vi "start.vi"(8 "error in (no error)":errorcluster, 11 "DL090202ScanHead in":refnum<class "ScanHeadDL090202.lvclass">) -> (0 "error out":errorcluster, 3 "DL090202ScanHead out":refnum<class "ScanHeadDL090202.lvclass">)   [LabVIEW 2010, in "ScanHeadDL090202.lvclass"]
uses:
  ScanHeadDL090202.lvclass
  SignalWriter/GenericSignalWriter/GenericSignalWriter/GenericSignalWriter.lvclass
  DAQ/GenericDAQ/GenericDAQ/GenericDAQ.lvclass
  Trajectory/GenericTrajectory/GenericTrajectory/GenericTrajectory.lvclass
  Clock/GenericClock/GenericClock/GenericClock.lvclass
  common/classes/ErrorController/ErrorController/ErrorController.lvclass
  DigitalOut/GenericDigitalOut/GenericDigitalOut/GenericDigitalOut.lvclass
  common/classes/GenericComponent/GenericComponent/GenericComponent.lvclass
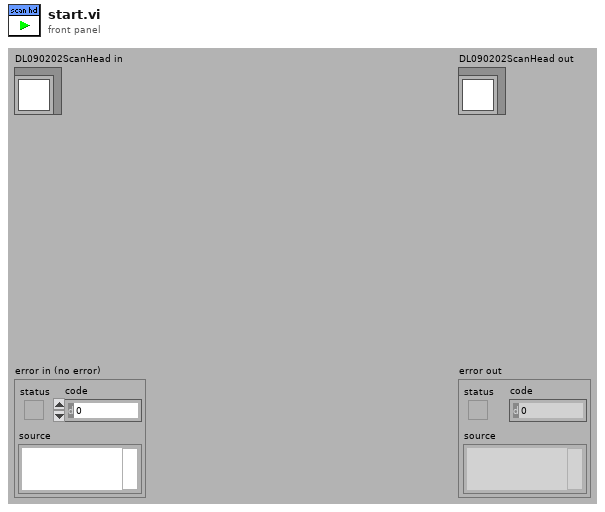
[diagram p1: front panel]
types:
  T1 = typedef "GenericToplevelComponent.lvclass/common_trigger_enum.ctl" = enum16{"NULL", "initialise", "terminate", "fetch command", "fetch data", "attach observer", "register as observer", "detach observer", "acknowledge", "start", "stop", "sweep started", "sweep finished", "experiment started", "experiment stopped"}
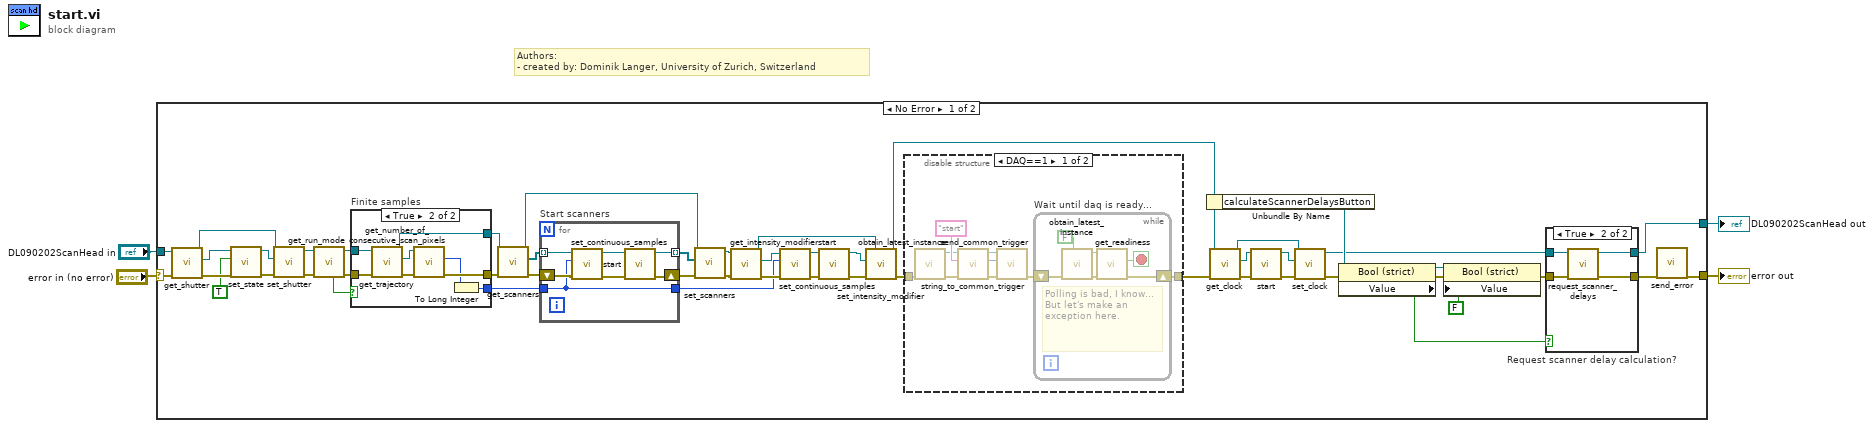
[diagram p0: block diagram]
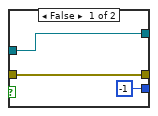
[diagram p4: hidden frame]
diagram:
  # "Authors: \n- created by: Dominik Langer, University of Zurich, Switzerland"
  n1 = case shown="No Error" "error in (no error)" {
    selector: "error in (no error)" -> [w21 w96]
    tunnel: [w10 w96] -> w3
    tunnel: [w5 w95] -> w1
    tunnel: "DL090202ScanHead in" -> [w22 w95]
    frame No Error {
      n2 = call-dynamic "get_shutter.vi"("error in (no error)"=w21, "DL090202ScanHead.lvclass in"=w22) -> ("error out"=w54:errorcluster, "GenericDigitalOut.lvclass"=w52:refnum<class "GenericDigitalOut.lvclass">, "DL090202ScanHead.lvclass out"=w51:refnum<class "ScanHeadDL090202.lvclass">)  [unwired: 7 out]
      n3 = call-dynamic "set_state.vi"("error in (no error)"=w54, "state"=TRUE, "GenericDigitalOut in"=w52) -> ("error out"=w53:errorcluster, "GenericDigitalOut out"=w50:refnum<class "GenericDigitalOut.lvclass">)  [unwired: 7 in]
      n4 = call-dynamic "set_shutter.vi"("error in (no error)"=w53, "GenericDigitalOut.lvclass"=w50, "DL090202ScanHead.lvclass in"=w51) -> ("error out"=w28:errorcluster, "DL090202ScanHead.lvclass out"=w29:refnum<class "ScanHeadDL090202.lvclass">)  [unwired: 7 out]
      n5 = call "get_run_mode.vi"("error in (no error)"=w28, "GenericPlugin in"=w29) -> ("error out"=w27:errorcluster, "GenericPlugin out"=w26:refnum<class "ScanHeadDL090202.lvclass">, "is NOT free run?"=w25:bool)  [unwired: 5 in, 2 out]
      n6 = case "Finite samples" shown="True" w25 {
        tunnel: [w79 w86] -> w33
        tunnel: [w78 w84] -> w32
        tunnel: [-1 w80] -> w31
        tunnel: w27 -> [w79 w83]
        tunnel: w26 -> [w78 w82]
        frame False {
        }
        frame True {
          n7 = call-dynamic "get_trajectory.vi"("error in (no error)"=w83, "GenericScanHead.lvclass in"=w82) -> ("error out"=w87:errorcluster, "trajectory"=w85:refnum<class "GenericTrajectory.lvclass">, "GenericScanHead.lvclass out"=w84:refnum<class "ScanHeadDL090202.lvclass">)  [unwired: 7 out]
          n8 = call-dynamic "get_number_of_consecutive_scan_pixels.vi"("error in (no error)"=w87, "GenericTrajectory in"=w85) -> ("error out"=w86:errorcluster, "number of consecutive scan pixels"=w81:i64)  [unwired: 8 out]
          n9 = To Long Integer(number=w81) -> (32bit integer=w80:i32)
        }
      }
      n10 = call-dynamic "get_scanners.vi"("error in (no error)"=w33, "DL090202ScanHead.lvclass in"=w32) -> ("error out"=w44:errorcluster, "scanners"=w43:refnum<class "GenericSignalWriter.lvclass">[], "DL090202ScanHead.lvclass out"=w7:refnum<class "ScanHeadDL090202.lvclass">)  [unwired: 7 out]
      n11 = for "Start scanners" {
        shift-right: [w94] -> w41
        shift-left: w44 -> [w92]
        tunnel: [w93] -> w39 mode=indexing
        tunnel: w43 -> [w90] mode=indexing
        tunnel: w31 -> [w88]
        tunnel: [w88] -> w30
        n12 = call-dynamic "set_continuous_samples.vi"("error in (no error)"=w92, "continuous samples"=w88, "GenericWriteSignals.lvclass in"=w90) -> ("error out"=w91:errorcluster, "GenericWriteSignals.lvclass out"=w89:refnum<class "GenericSignalWriter.lvclass">)  [unwired: 7 out]
        n13 = call-dynamic "start.vi"("error in (no error)"=w91, "WriteSignalsGenericPlugin in"=w89) -> ("error out"=w94:errorcluster, "WriteSignalsGenericPlugin out"=w93:refnum<class "GenericSignalWriter.lvclass">)  [unwired: 8 out]
      }
      n14 = call-dynamic "set_scanners.vi"("error in (no error)"=w41, "scanners"=w39, "DL090202ScanHead.lvclass in"=w7) -> ("error out"=w42:errorcluster, "DL090202ScanHead.lvclass out"=w38:refnum<class "ScanHeadDL090202.lvclass">)  [unwired: 7 out]
      n15 = call-dynamic "get_intensity_modifier.vi"("error in (no error)"=w42, "DL090202ScanHead.lvclass in"=w38) -> ("error out"=w40:errorcluster, "write signals"=w35:refnum<class "GenericSignalWriter.lvclass">, "DL090202ScanHead.lvclass out"=w34:refnum<class "ScanHeadDL090202.lvclass">)  [unwired: 7 out]
      n16 = call-dynamic "set_continuous_samples.vi"("error in (no error)"=w40, "continuous samples"=w30, "GenericWriteSignals.lvclass in"=w35) -> ("error out"=w12:errorcluster, "GenericWriteSignals.lvclass out"=w11:refnum<class "GenericSignalWriter.lvclass">)  [unwired: 7 out]
      n17 = call-dynamic "start.vi"("error in (no error)"=w12, "WriteSignalsGenericPlugin in"=w11) -> ("error out"=w37:errorcluster, "WriteSignalsGenericPlugin out"=w36:refnum<class "GenericSignalWriter.lvclass">)  [unwired: 8 out]
      n18 = call-dynamic "set_intensity_modifier.vi"("error in (no error)"=w37, "write signals"=w36, "DL090202ScanHead.lvclass in"=w34) -> ("error out"=w23:errorcluster, "DL090202ScanHead.lvclass out"=w8:refnum<class "ScanHeadDL090202.lvclass">)  [unwired: 7 out]
      n19 = disable-structure shown="DAQ==1" {
        disable-tunnel: [w69 w76] -> w24
        disable-tunnel: w23 -> [w67 w76]
        frame condition #0 {
          n20 = call "obtain_latest_instance.vi"("error in (no error)"=w67) -> ("error out"=w64:errorcluster, "GenericDAQ out"=w65:refnum<class "GenericDAQ.lvclass">)  [unwired: 9 in]
          n21 = call-dynamic "string_to_common_trigger.vi"("error in (no error)"=w64, "trigger string"="start", "GenericToplevelComponent in"=w65) -> ("error out"=w63:errorcluster, "trigger"=w61:T1, "GenericToplevelComponent out"=w62:refnum<class "GenericDAQ.lvclass">)  [unwired: 6 in]
          n22 = call-dynamic "send_common_trigger.vi"("error in (no error)"=w63, "trigger"=w61, "GenericToplevelComponent in"=w62) -> ("error out"=w68:errorcluster)  [unwired: 6 in, 2 out]
          n23 = while "Wait until daq is ready..." {
            shift-right: [w71] -> w69
            shift-left: w68 -> [w72]
            stop <- w70 stop-if-true
            # "Polling is bad, I know...\nBut let's make an exception here."
            n24 = call "obtain_latest_instance.vi"("quick, but maybe outdated?"=FALSE, "error in (no error)"=w72) -> ("error out"=w75:errorcluster, "GenericDAQ out"=w74:refnum<class "GenericDAQ.lvclass">)  [unwired: 8 in]
            n25 = call-dynamic "get_readiness.vi"("error in (no error)"=w75, "GenericDAQ in"=w74) -> ("error out"=w71:errorcluster, "ready?"=w70:bool)  [unwired: 7 in, 1 out]
          }
        }
        frame condition #1 (active) {
        }
      }
      n26 = Unbundle By Name(w8) -> ("calculateScannerDelaysButton"=w16:refnum<vi>)
      n27 = call-dynamic "get_clock.vi"("error in (no error)"=w24, "DL090202ScanHead.lvclass in"=w8) -> ("error out"=w49:errorcluster, "GenericClock.lvclass"=w48:refnum<class "GenericClock.lvclass">, "DL090202ScanHead.lvclass out"=w45:refnum<class "ScanHeadDL090202.lvclass">)  [unwired: 7 out]
      n28 = call-dynamic "start.vi"("error in (no error)"=w49, "GenericClock in"=w48) -> ("error out"=w47:errorcluster, "GenericClock out"=w46:refnum<class "GenericClock.lvclass">)  [unwired: 8 out]
      n29 = call-dynamic "set_clock.vi"("error in (no error)"=w47, "GenericClock.lvclass"=w46, "DL090202ScanHead.lvclass in"=w45) -> ("error out"=w18:errorcluster, "DL090202ScanHead.lvclass out"=w13:refnum<class "ScanHeadDL090202.lvclass">)  [unwired: 7 out]
      n30 = property class="Bool (strict)"(reference=w16, error in=w18) -> (reference out=w15:refnum<vi>, error out=w17:errorcluster, "Value"=w19:bool)
      n31 = property class="Bool (strict)"(reference=w15, error in=w17, "Value"=FALSE) -> (error out=w14:errorcluster)  [unwired: 1 out]
      n32 = case "Request scanner delay calculation?" shown="True" w19 {
        tunnel: w14 -> [w56 w60]
        tunnel: [w56 w59] -> w6
        tunnel: w13 -> [w55 w58]
        tunnel: [w55 w57] -> w5
        frame False {
        }
        frame True {
          n33 = call-dynamic "request_scanner_delays.vi"("error in (no error)"=w60, "ScanHeadDL090202 in"=w58) -> ("error out"=w59:errorcluster, "ScanHeadDL090202 out"=w57:refnum<class "ScanHeadDL090202.lvclass">)  [unwired: 8 in]
        }
      }
      n34 = call "send_error.vi"("error in (no error)"=w6) -> ("error out"=w10:errorcluster)  [unwired: 10 in]
    }
    frame Error {
    }
  }
  "error out" <- w3
  "DL090202ScanHead out" <- w1
